vi "exitingCurrentState.vi"(8 "error in (no error)":errorcluster, 11 "statemachine in":refnum<class "statemachine.lvclass">) -> (0 "error out":errorcluster, 3 "statemachine out":refnum<class "statemachine.lvclass">)   [LabVIEW 2020, in "eos.lvlib" / "statemachine.lvclass"]
uses:
  statemachine.lvclass
  interfaces/state/state.lvclass
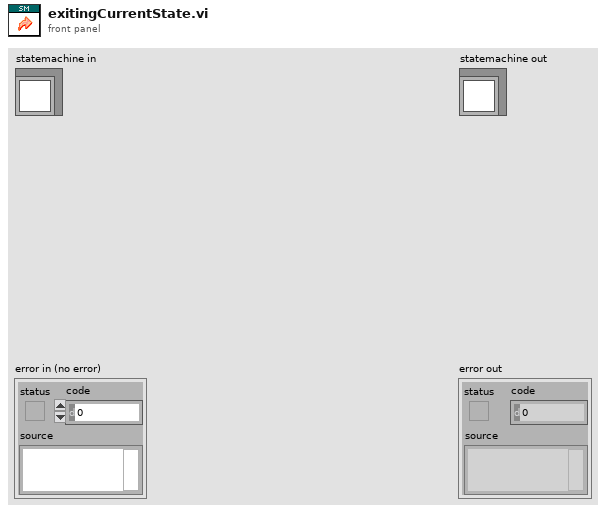
[diagram p1: front panel]
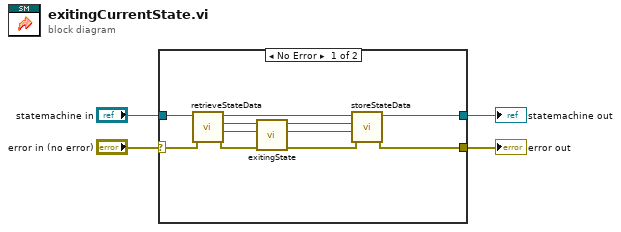
[diagram p0: block diagram]
diagram:
  n1 = case shown="No Error" "error in (no error)" {
    selector: "error in (no error)" -> [w7 w17]
    tunnel: [w13 w17] -> w3
    tunnel: [w15 w16] -> w1
    tunnel: "statemachine in" -> [w9 w16]
    frame No Error {
      n2 = call "retrieveStateData.vi"("error in (no error)"=w7, "statemachine in"=w9) -> ("error out"=w8:errorcluster, "State Data"=w12:refnum<class "data.lvclass">, "State"=w6:refnum<class "state.lvclass">, "statemachine out"=w10:refnum<class "statemachine.lvclass">)  [unwired: 6 in]
      n3 = call-dynamic "exitingState.vi"("error in (no error)"=w8, "State Data in"=w12, "State in"=w6) -> ("error out"=w14:errorcluster, "State Data out"=w11:refnum<class "data.lvclass">, "State out"=w5:refnum<class "state.lvclass">)  [unwired: 6 in]
      n4 = call "storeStateData.vi"("error in (no error)"=w14, "State Data"=w11, "Current State"=w5, "statemachine in"=w10) -> ("error out"=w13:errorcluster, "statemachine out"=w15:refnum<class "statemachine.lvclass">)  [unwired: 5 in, 1 out]
    }
    frame Error {
    }
  }
  "error out" <- w3
  "statemachine out" <- w1
